vi "Set FPGA Props and Dependencies.vi"(7 "VS FPGA?":bool, 8 "error in (no error)":errorcluster, 9 "FPGA Ref":T1 format="%.0x", 10 "CD Ref in":T1 format="%.0x", 11 "Win User BF Path":path) -> (0 "error out":errorcluster, 3 "CD Ref out":T1 format="%.0x")   [LabVIEW 2011, in "Engine Sim System Explorer.lvlib"]
uses:
  Engine Sim System Explorer.lvlib
  <vilib>/NI Veristand/Custom Device API/Custom Device Item Ref.ctl
  <vilib>/NI Veristand/Custom Device API/Dependent File Optional Info.ctl
  Shared/Engine Simulation Global.vi
  <vilib>/NI Veristand/Custom Device API/Set Item Property (Path).vi
  <vilib>/NI Veristand/Custom Device API/Set Item Property (Boolean).vi
  <vilib>/NI Veristand/Custom Device API/Set Item Property (Dependent Node Pointer).vi
  <vilib>/NI Veristand/Custom Device API/Set Item Property (Dependent File).vi
  <vilib>/NI Veristand/Custom Device API/Custom Device API.lvlib
  Engine Simulation Shared.lvlib
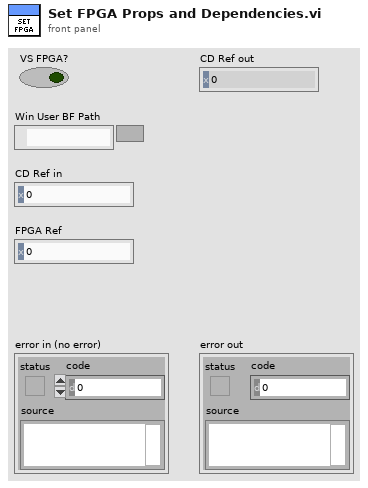
[diagram p1: front panel]
types:
  T1 = typedef "Custom Device API.lvlib/Custom Device Item Ref.ctl" = u64
  T2 = typedef "Custom Device API.lvlib/Dependent File Optional Info.ctl" = cluster{"Version":string, "RTDestination":path, "ForceDownload":bool, "SupportedTarget":string, "MD5":string}
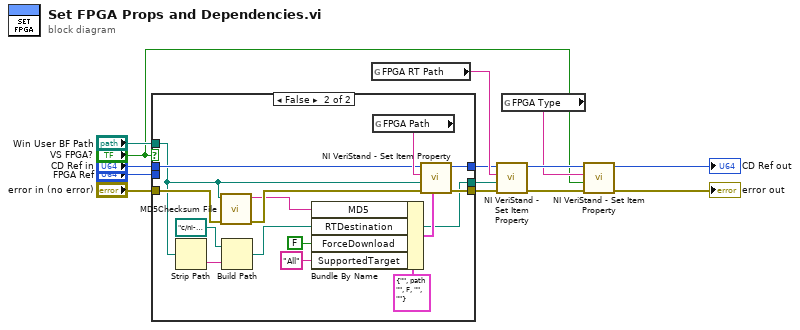
[diagram p0: block diagram]
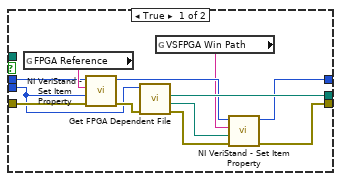
[diagram p2: hidden frame]
diagram:
  n1 = case shown="False" "VS FPGA?" {
    tunnel: "FPGA Ref" -> [w22 _]
    tunnel: "error in (no error)" -> [w24 w30]
    tunnel: "CD Ref in" -> [w25 w40]
    tunnel: "Win User BF Path" -> [_ w27]
    tunnel: [w19 w39] -> w11
    tunnel: [w17 w38] -> w12
    tunnel: [w21 w31] -> w13
    frame True {
      n2 = global read "Engine Simulation Global.vi" "FPGA Reference"() -> (w26:string)
      n3 = call-poly <vilib>:"NI VeriStand - Set Item Property.vi"("error in (no error)"=w24, "Dependent Node Ref"=w22, "Property Name"=w26, "Item Ref in"=w25) -> ("error out"=w23:errorcluster, "Item Ref out"=w18:T1)  [unwired: 5 in, 1 out]
      n4 = call "Get FPGA Dependent File.vi"("error in (no error)"=w23, "ID in"=w22) -> ("error out"=w20:errorcluster, "Windows Path"=w16:path, "RT Path"=w21:path)  [unwired: 6 in, 1 out]
      n5 = global read "Engine Simulation Global.vi" "VSFPGA Win Path"() -> (w15:string)
      n6 = call-poly <vilib>:"NI VeriStand - Set Item Property.vi"("error in (no error)"=w20, "Value"=w16, "Property Name"=w15, "Item Ref in"=w18) -> ("error out"=w19:errorcluster, "Item Ref out"=w17:T1)  [unwired: 5 in, 1 out]
    }
    frame False {
      n7 = Strip Path(path=w27) -> (name=w37:string)  [unwired: 1 out]
      n8 = call <vilib>:"MD5Checksum File.vi"("error in (no error)"=w30, "Path"=w27) -> ("error out"=w29:errorcluster, "MD5 message-digest"=w28:string)  [unwired: 8 in]
      n9 = Build Path(base path=path "c:/ni-rt/NIVeriStand/Custom Devices/Engine Simulation" ("RTDestination"), name or relative path=w37) -> (appended path=w31:path)
      n10 = Bundle By Name(cluster=T2 {"Version"="", "RTDestination"=path "", "ForceDownload"=FALSE, "SupportedTarget"="", "MD5"=""} ("OptionalInfo"), "MD5"=w28, "RTDestination"=w31, "ForceDownload"=FALSE, "SupportedTarget"="All") -> (w33:T2)
      n11 = global read "Engine Simulation Global.vi" "FPGA Path"() -> (w41:string)
      n12 = call-poly <vilib>:"NI VeriStand - Set Item Property.vi"("OptionalInfo"=w33, "error in (no error)"=w29, "Path"=w27, "Property Name"=w41, "Item Ref in"=w40) -> ("error out"=w39:errorcluster, "Item Ref out"=w38:T1)  [unwired: 4 in, 1 out]
    }
  }
  n13 = global read "Engine Simulation Global.vi" "FPGA RT Path"() -> (w14:string)
  n14 = call-poly <vilib>:"NI VeriStand - Set Item Property.vi"("error in (no error)"=w11, "Value"=w13, "Property Name"=w14, "Item Ref in"=w12) -> ("error out"=w6:errorcluster, "Item Ref out"=w5:T1)  [unwired: 5 in, 1 out]
  n15 = global read "Engine Simulation Global.vi" "FPGA Type"() -> (w2:string)
  n16 = call-poly <vilib>:"NI VeriStand - Set Item Property.vi"("error in (no error)"=w6, "Value"="VS FPGA?", "Property Name"=w2, "Item Ref in"=w5) -> ("error out"=→"error out":errorcluster, "Item Ref out"=→"CD Ref out":T1)  [unwired: 5 in, 1 out]
